vi "KeyValue2Pair.vi"(10 "值":string, 11 "键":string) -> (3 "键值对":string)   [LabVIEW 2020, in "Curve Editor.lvlib" / "Key Value.lvlib"]
uses:
  Key Value.lvlib
panel:
  # "将键和值组合成键值对"
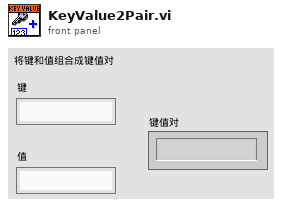
[diagram p1: front panel]
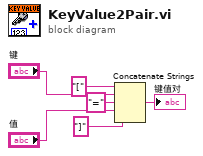
[diagram p0: block diagram]
diagram:
  n1 = Concatenate Strings("[" ("字符串"), "键", "=" ("字符串"), "值", "]" ("字符串")) -> (→"键值对":string)
